vi "acq.Stop.vi"(0 "DVR":T1) -> ()   [LabVIEW 2020]
uses:
  _controls/data.ctl
  camera/camera.lvclass
  _controls/data.ref.ctl
  <vilib>/vision/Image Controls.llb/IMAQ Image.ctl
  _controls/state.ctl
  _controls/data.vars.ctl
  _controls/save_options.ctl
  _controls/flip.ctl
  f9d285f5-898e-47b3-ab9c-5e55c0ecfd4d.vi
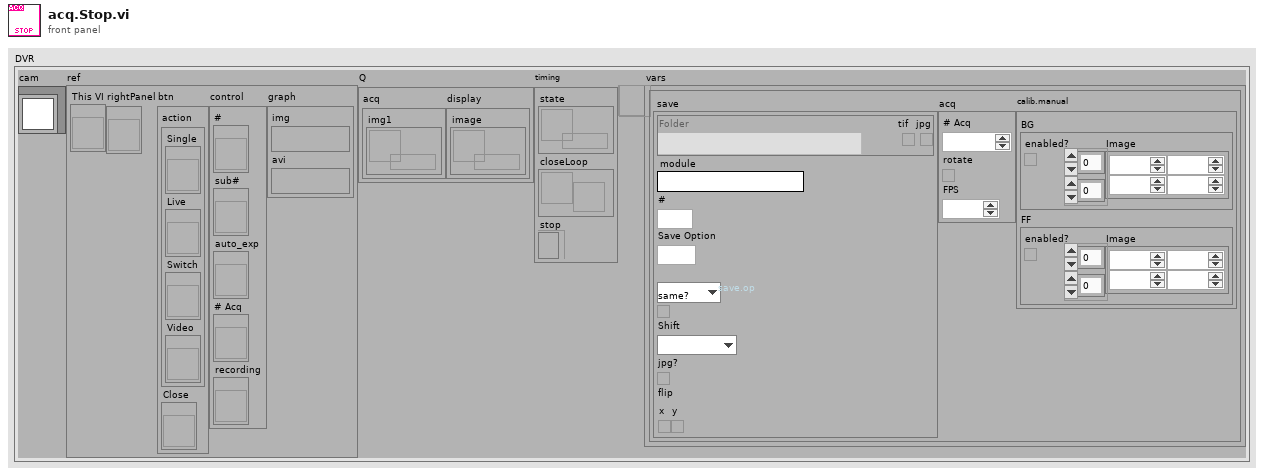
[diagram p1: front panel]
types:
  T1 = typedef "data.ctl" = cluster{"cam":refnum<class "camera.lvclass">, "ref":T2, "Q":cluster{"acq":cluster{"img1":refnum<queue>}, "display":cluster{"image":refnum<queue>}}, "timing":cluster{"state":refnum<queue>, "closeLoop":refnum<notifier>, "stop":refnum<k4>}, "vars":refnum<data-value>}
  T2 = typedef "data.ref.ctl" = cluster{"This VI":refnum<vi>, "rightPanel":refnum<vi>, "btn":cluster{"action":cluster{"Single":refnum<vi>, "Live":refnum<vi>, "Switch":refnum<vi>, "Video":refnum<vi>}, "Close":refnum<vi>}, "control":cluster{"#":refnum<vi>, "sub#":refnum<vi>, "auto_exp":refnum<vi>, "# Acq":refnum<vi>, "recording":refnum<vi>}, "graph":cluster{"img":T3, "avi":T3}}
  T3 = typedef "IMAQ Image.ctl" = refnum<image>
  T4 = typedef "state.ctl" = enum16{"-", "single", "video", "livePL", "PL"}
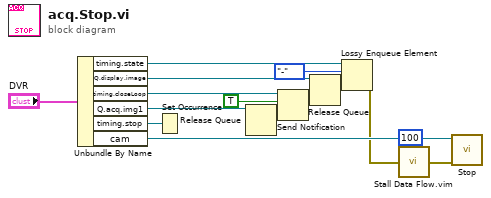
[diagram p0: block diagram]
diagram:
  n1 = Unbundle By Name("DVR") -> ("timing.state"=w10:refnum<queue>, "Q.display.image"=w7:refnum<queue>, "timing.closeLoop"=w9:refnum<notifier>, "Q.acq.img1"=w5:refnum<queue>, "timing.stop"=w12:refnum<k4>, "cam"=w4:refnum<class "camera.lvclass">)
  n2 = Set Occurrence(w12) -> ()
  n3 = Release Queue(queue=w5) -> ()  [unwired: 2 in, 3 out]
  n4 = Send Notification(notification=TRUE, notifier=w9) -> ()  [unwired: 1 in, 2 out]
  n5 = Release Queue(queue=w7) -> ()  [unwired: 2 in, 3 out]
  n6 = Lossy Enqueue Element(queue=w10, element=state."-") -> (error out=w3:errorcluster)  [unwired: 1 in, 3 out]
  n7 = call "Stall Data Flow.vim"("value in"=w3, "milliseconds to wait"=u32 100) -> ("value out"=w2:errorcluster)  [unwired: 1 out]
  n8 = call-dynamic "Stop.vi"("error in"=w2, "camera.nit in"=w4) -> ()  [unwired: 9 in, 1 out]
